vi "AgilentAndNiDmm.vi"() -> ()   [LabVIEW 2014]
uses:
  <instrlib>/niDMM/nidmm.llb/niDMM Slope.ctl
  <instrlib>/niDMM/nidmm.llb/niDMM Trigger.ctl
  <instrlib>/niDMM/nidmm.llb/niDMM Resolution in Digits.ctl
  <instrlib>/niDMM/nidmm.llb/niDMM Function.ctl
  <vilib>/Utility/error.llb/DialogType.ctl
  <instrlib>/niDMM/nidmm.llb/niDMM Sample Trigger.ctl
  <instrlib>/niDMM/nidmm.llb/niDMM Configure Measurement Digits.vi
  <instrlib>/Agilent 34401/Agilent 34401.lvlib
panel:
  out "Actual Number to fetch":i32 caption="Actual Number"
  out "Dif: NiDmm - Agilent":dbl[](graph)=[0.002500734, 0.002496723, 0.002491019, 0.002484271, 0.002477294]
  out "Measurements":dbl[](graph)
  in  "Function (0: DC Voltage)":u16(ring) items=["DC Voltage", "AC Voltage", "2 - Wire Resistance", "4 - Wire Resistance", "DC Current", "AC Current", "Frequency", "Period", "Continuity", "Diode Checking", "VDC:VDC Ratio", "Temperature", "Capacitance"]
  in  "Trigger Source (0: Immediate)":u16(ring) items=["Immediate", "Software (Bus)", "External", "Internal"]
  in  "Manual Range (1.00)":dbl=1.0 format="%_3f"
  in  "Enable Auto Range (F: Disable)":bool
  in  "Trigger Count (5)":i32=5 format="%#.6g"
  out "Measurements 2":dbl[](graph)=[0.002500734, 0.002496723, 0.002491019, 0.002484271, 0.002477294]
  out "Trigger Iteration":i32
  in  "Stop":bool
  in  "Samples per Trigger (10)":i32=10 format="%#.6g"
  in  "Timeout (10000 ms)":u32=10000
  in  "VISA resource name":refnum<visa-resource-name>
  in  "Function":T1
  in  "Resolution in Digits":T2=5.5 items=["3 1/2"=3.5, "4 1/2"=4.5, "5 1/2"=5.5, "6 1/2"=6.5, "7 1/2"=7.5]
  in  "Range":dbl=10.0 format="%.2p"
  in  "Trigger Source":T3=enum."External"
  in  "Slope":T4=enum."Falling Edge"
  in  "Device Name":refnum<k15>="Dev1"
  # "NI DMM"
  # "AGILENT"
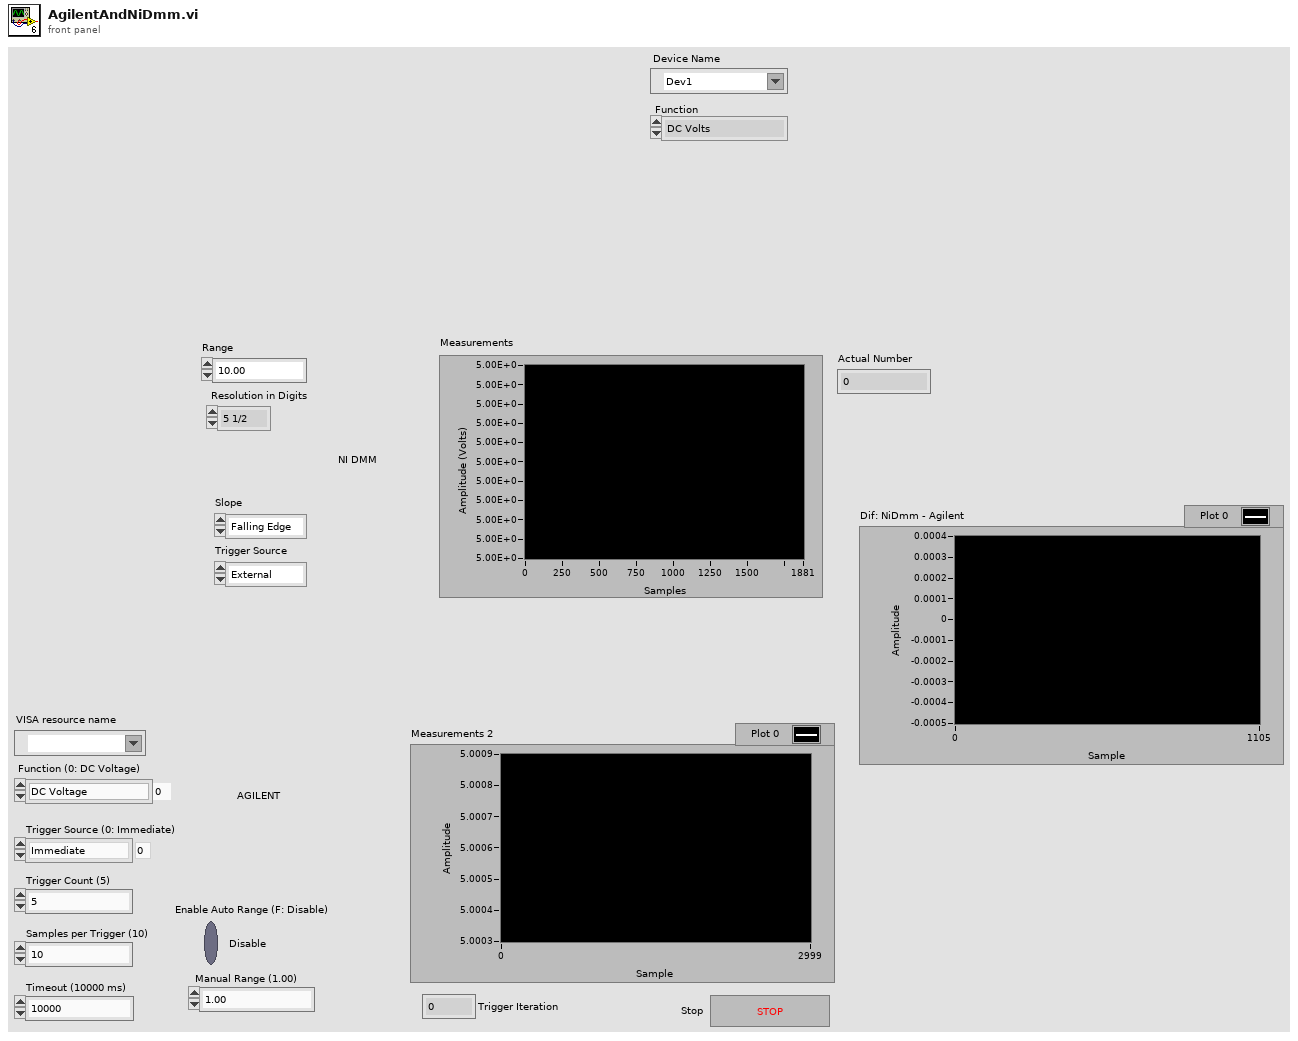
[diagram p1: front panel]
types:
  T1 = typedef "niDMM Function.ctl" = enum16{"DC Volts", "AC Volts", "DC Current", "AC Current", "2-wire Resistance", "4-wire Resistance", "Diode", "Frequency", "Period", "AC Volts DC Coupled", "Capacitance", "Inductance", "Temperature"}
  T2 = typedef "niDMM Resolution in Digits.ctl" = dbl
  T3 = typedef "niDMM Trigger.ctl" = enum16{"Immediate", "External", "TTL 0", "TTL 1", "TTL 2", "TTL 3", "TTL 4", "TTL 5", "TTL 6", "Software", "TTL 7", "PXI Star", "LBR Trig 1", "Aux Trig 1"}
  T4 = typedef "niDMM Slope.ctl" = enum16{"Rising Edge", "Falling Edge"}
  T5 = typedef "DialogType.ctl" = u16
  T6 = typedef "niDMM Sample Trigger.ctl" = enum16{"Immediate", "External", "TTL 0", "TTL 1", "TTL 2", "TTL 3", "TTL 4", "TTL 5", "TTL 6", "Interval", "Software", "TTL 7", "PXI Star", "LBR Trig 1", "Aux Trig 1"}
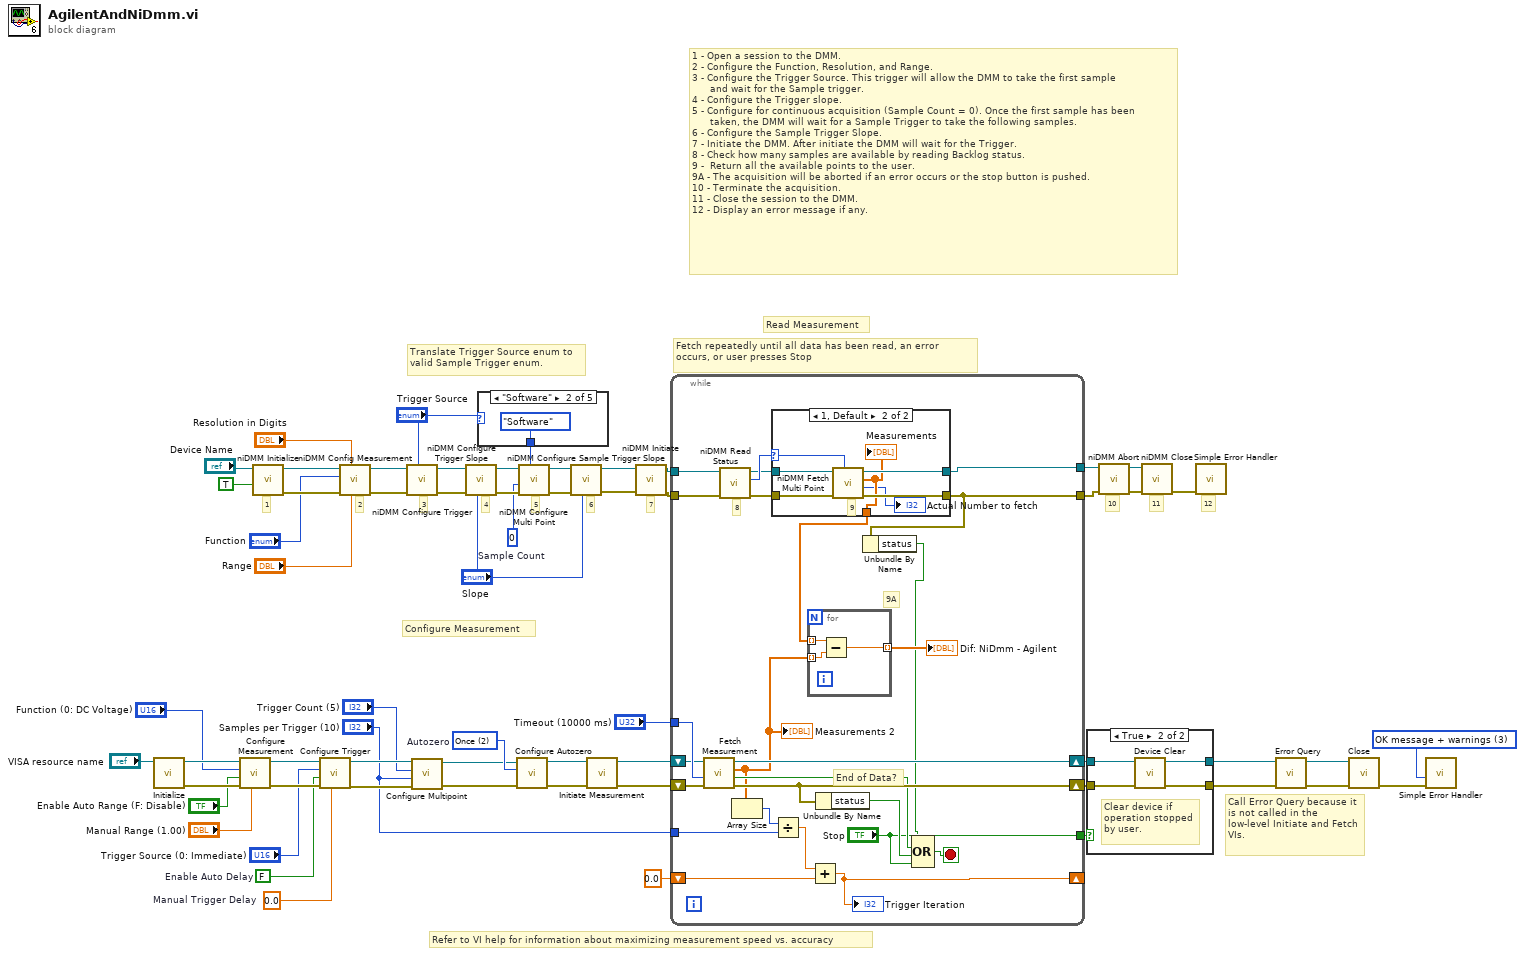
[diagram p0: block diagram]
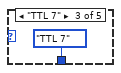
[diagram p5: hidden frame]
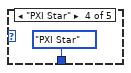
[diagram p6: hidden frame]
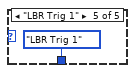
[diagram p7: hidden frame]
diagram:
  w7 = 0.0  # Manual Trigger Delay
  w8 = FALSE  # Enable Auto Delay
  w16 = T5 3 items=["no dialog", "OK message", "continue or stop message", "OK message + warnings", "continue/stop + warnings"] ("type of dialog (OK msg:1)")
  w34 = u16 2 items=["On", "Off", "Once"]  # Autozero
  w47 = 0  # Sample Count
  # "Call Error Query because it is not called in the low-level Initiate and Fetch VIs."
  # "Fetch repeatedly until all data has been read, an error occurs, or user presses Stop"
  # "Refer to VI help for information about maximizing measurement speed vs. accuracy"
  # "Read Measurement"
  # "Configure Measurement"
  # "4"
  # "12"
  # "10"
  # "6"
  # "11"
  # "5"
  # "7"
  # "Translate Trigger Source enum to\nvalid Sample Trigger enum."
  # "3"
  # "2"
  # "1"
  # "1 - Open a session to the DMM.\n2 - Configure the Function, Resolution, and Range.\n3 - Configure the Trigger Source. This trigger will allow the DMM to take the first sample\n      and wait for the Sample trigger.\n4 - Configure the Trigger slope.\n5 - Configure for continuous acquisition (Sample Count = 0). Once the first sample has been\n      taken, the DMM will wait for a Sample Trigger to take the following samples.\n6 - Configure the Sample Trigger Slope.\n7 - Initiate the DMM. After initiate the DMM will wait for the Trigger.\n8 - Check how many samples are available by reading Backlog status.  \n9 -  Return all the available points to the user. \n9A - The acquisition will be aborted if an error occurs or the stop button is pushed.\n10 - Terminate the acquisition.\n11 - Close the session to the DMM.\n12 - Display an error message if any."
  n1 = call <instrlib>:"Initialize.vi"("VISA resource name"="VISA resource name") -> ("error out"=w35:errorcluster, "VISA resource name out"=w36:refnum<visa-resource-name>)  [unwired: 9 in]
  n2 = call <instrlib>:"Configure Measurement.vi"("Manual Range (1.00)"="Manual Range (1.00)", "error in (no error)"=w35, "Enable Auto Range (T: Enable)"="Enable Auto Range (F: Disable)", "Function (0: DC Voltage)"="Function (0: DC Voltage)", "VISA resource name"=w36) -> ("error out"=w27:errorcluster, "VISA resource name out"=w28:refnum<visa-resource-name>)  [unwired: 5 in]
  n3 = call <instrlib>:"niDMM Initialize.vi"("Reset"=TRUE, "Instrument Descriptor"="Device Name") -> ("error out"=w60:errorcluster, "instrument handle out"=w61:refnum<k15>)  [unwired: 8 in]
  n4 = call <instrlib>:"Configure Trigger.vi"("Manual Trigger Delay (0.0 s)"=w7, "error in (no error)"=w27, "Enable Auto Delay (T: Enable)"=w8, "Trigger Source (0: Immediate)"="Trigger Source (0: Immediate)", "VISA resource name"=w28) -> ("error out"=w25:errorcluster, "VISA resource name out"=w26:refnum<visa-resource-name>)  [unwired: 5 in]
  n5 = call-poly <instrlib>:"niDMM Config Measurement.vi"("Range"="Range", "Resolution in Digits"="Resolution in Digits", "error in (no error)"=w60, "Function"="Function", "instrument handle"=w61) -> ("error out"=w54:errorcluster, "instrument handle out"=w55:refnum<k15>)  [unwired: 5 in]
  n6 = call <instrlib>:"niDMM Configure Trigger.vi"("Trigger Source"="Trigger Source", "error in (no error)"=w54, "instrument handle"=w55) -> ("error out"=w52:errorcluster, "instrument handle out"=w53:refnum<k15>)  [unwired: 7 in]
  n7 = call <instrlib>:"Configure Multipoint.vi"("error in (no error)"=w25, "Sample Count (1)"="Samples per Trigger (10)", "Trigger Count (1)"="Trigger Count (5)", "VISA resource name"=w26) -> ("error out"=w31:errorcluster, "VISA resource name out"=w32:refnum<visa-resource-name>)  [unwired: 6 in]
  n8 = call <instrlib>:"niDMM Configure Trigger Slope.vi"("Slope"="Slope", "error in (no error)"=w52, "instrument handle"=w53) -> ("error out"=w50:errorcluster, "instrument handle out"=w51:refnum<k15>)  [unwired: 7 in]
  n9 = case shown="\"Software\"" "Trigger Source" {
    selector: "Trigger Source" -> [w62 _ _ _ _]
    tunnel: [w62 niDMM_Sample_Trigger."Software" ("Sample Trigger") niDMM_Sample_Trigger."TTL 7" ("Sample Trigger") niDMM_Sample_Trigger."PXI Star" ("Sample Trigger") niDMM_Sample_Trigger."LBR Trig 1" ("Sample Trigger")] -> w43
    frame "Immediate", Default {
    }
    frame "Software" {
    }
    frame "TTL 7" {
    }
    frame "PXI Star" {
    }
    frame "LBR Trig 1" {
    }
  }
  n10 = call <instrlib>:"Configure Autozero.vi"("error in (no error)"=w31, "Autozero  (0: On)"=w34, "VISA resource name"=w32) -> ("error out"=w23:errorcluster, "VISA resource name out"=w24:refnum<visa-resource-name>)  [unwired: 7 in]
  n11 = call <instrlib>:"niDMM Configure Multi Point.vi"("Sample Trigger"=w43, "error in (no error)"=w50, "Sample Count"=w47, "instrument handle"=w51) -> ("error out"=w1:errorcluster, "instrument handle out"=w49:refnum<k15>)  [unwired: 6 in]
  n12 = call <instrlib>:"niDMM Configure Sample Trigger Slope.vi"("Slope"="Slope", "error in (no error)"=w1, "instrument handle"=w49) -> ("error out"=w45:errorcluster, "instrument handle out"=w42:refnum<k15>)  [unwired: 7 in]
  n13 = call <instrlib>:"Initiate Measurement.vi"("error in (no error)"=w23, "VISA resource name"=w24) -> ("error out"=w21:errorcluster, "VISA resource name out"=w22:refnum<visa-resource-name>)  [unwired: 8 in]
  n14 = call <instrlib>:"niDMM Initiate.vi"("error in (no error)"=w45, "instrument handle"=w42) -> ("error out"=w3:errorcluster, "instrument handle out"=w4:refnum<k15>)  [unwired: 8 in]
  n15 = while {
    tunnel: "Timeout (10000 ms)" -> [w90]
    shift-right: [w86] -> w29
    shift-left: w21 -> [w88]
    shift-right: [w91] -> w30
    shift-left: w22 -> [w89]
    tunnel: ["Stop"] -> w20
    tunnel: "Samples per Trigger (10)" -> [w81]
    shift-right: [w79] -> _
    shift-left: 0.0 -> [w78]
    tunnel: [w74] -> w5
    tunnel: w4 -> [w73]
    tunnel: w3 -> [w72]
    tunnel: [w71] -> w2
    stop <- w87 stop-if-true
    # "9A"
    # "8"
    # "End of Data?"
    n16 = call <instrlib>:"Fetch Measurement.vi"("error in (no error)"=w88, "Timeout (10000 ms)"=w90, "VISA resource name"=w89) -> ("error out"=w86:errorcluster, "End of Data?"=w84:bool, "Measurements"=w69:dbl[], "VISA resource name out"=w91:refnum<visa-resource-name>)  [unwired: 5 in]
    "Measurements 2" <- w69
    n17 = call <instrlib>:"niDMM Read Status.vi"("error in (no error)"=w72, "instrument handle"=w73) -> ("error out"=w75:errorcluster, "Backlog"=w77:i32, "instrument handle out"=w76:refnum<k15>)  [unwired: 6 in, 1 out]
    n18 = Array Size(array=w69) -> (size(s)=w82:i32)
    n19 = case shown="1, Default" w77 {
      selector: w77 -> [_ w99]
      tunnel: [w96 w103] -> w74
      tunnel: [w95 w102] -> w71
      tunnel: w75 -> [w95 w101]
      tunnel: w76 -> [w96 w100]
      tunnel: [_ w98] -> w70
      frame 0 {
      }
      frame 1, Default {
        # "9"
        n20 = call <instrlib>:"niDMM Fetch Multi Point.vi"("Number to Fetch"=w99, "error in (no error)"=w101, "instrument handle"=w100) -> ("error out"=w102:errorcluster, "Actual Number"=→"Actual Number to fetch":i32, "Measurements"=w98:dbl[], "instrument handle out"=w103:refnum<k15>)  [unwired: 5 in]
        "Measurements" <- w98
      }
    }
    n21 = Divide(x=w82, y=w81) -> (x/y=w80:dbl)
    n22 = for {
      tunnel: w70 -> [w94] mode=indexing
      tunnel: w69 -> [w93] mode=indexing
      tunnel: [w92] -> w68 mode=indexing
      n23 = Subtract(x=w94, y=w93) -> (x-y=w92:dbl)
    }
    "Dif: NiDmm - Agilent" <- w68
    n24 = Add(x=w80, y=w78) -> (x+y=w79:dbl)
    "Trigger Iteration" <- w79
    n25 = Unbundle By Name(w86) -> ("status"=w85:bool)
    n26 = Unbundle By Name(w71) -> ("status"=w67:bool)
    n27 = Compound Arithmetic op=OR(w67, w84, w85, "Stop") -> (w87:bool)
  }
  n28 = case shown="True" w20 {
    tunnel: w30 -> [w105 w109]
    tunnel: w29 -> [w104 w108]
    tunnel: [w105 w107] -> w11
    tunnel: [w104 w106] -> w10
    frame False {
    }
    frame True {
      # "Clear device if operation stopped by user."
      n29 = call <instrlib>:"Device Clear.vi"("error in (no error)"=w108, "VISA Resource Name"=w109) -> ("error out"=w106:errorcluster, "VISA Resource Out"=w107:refnum<visa-resource-name>)  [unwired: 8 in]
    }
  }
  n30 = call <instrlib>:"niDMM Abort.vi"("error in (no error)"=w2, "instrument handle"=w5) -> ("error out"=w58:errorcluster, "instrument handle out"=w59:refnum<k15>)  [unwired: 8 in]
  n31 = call <instrlib>:"niDMM Close.vi"("error in (no error)"=w58, "instrument handle"=w59) -> ("error out"=w41:errorcluster)  [unwired: 9 in]
  n32 = call <vilib>:"Simple Error Handler.vi"("error in (no error)"=w41) -> ()  [unwired: 4 in, 5 out]
  n33 = call <instrlib>:"Error Query.vi"("error in (no error)"=w10, "VISA resource name"=w11) -> ("error out"=w13:errorcluster, "VISA resource name out"=w12:refnum<visa-resource-name>)  [unwired: 6 in, 2 out]
  n34 = call <instrlib>:"Close.vi"("error in (no error)"=w13, "VISA resource name"=w12) -> ("error out"=w38:errorcluster)  [unwired: 9 in]
  n35 = call <vilib>:"Simple Error Handler.vi"("type of dialog (OK msg:1)"=w16, "error in (no error)"=w38) -> ()  [unwired: 3 in, 5 out]
